vi "Register for Events (Cluster).vi"(8 "error in (no error)":errorcluster, 9 "Object":T1, 11 "JKI_Python_Server in":refnum<class "Server.lvclass">) -> (0 "error out":errorcluster, 1 "Python":T2, 3 "JKI_Python_Server out":refnum<class "Server.lvclass">)   [LabVIEW 2013, in "JKI_Python_Bridge_for_LV.lvlib" / "Server.lvclass"]
uses:
  Server.lvclass
  Type Definitions/Python Method Call - Event Registration.ctl
  Call/Call.lvclass
  Type Definitions/Public Events - Cluster.ctl
  CallHandler/PyObject.lvclass
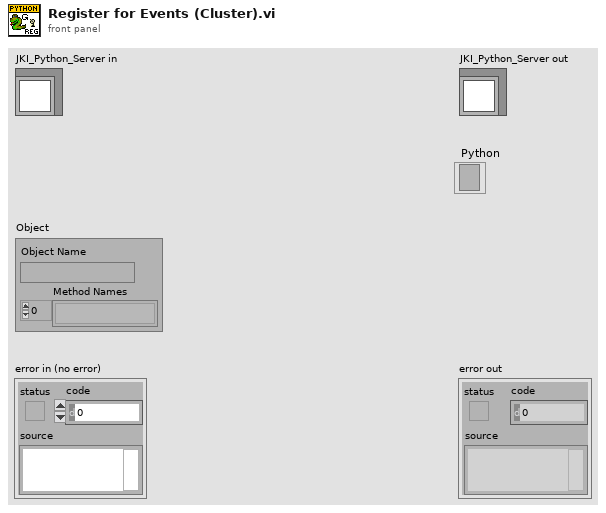
[diagram p1: front panel]
types:
  T1 = cluster{"Object Name":string, "Method Names":string[]}
  T2 = typedef "JKI_Python_Bridge_for_LV.lvlib/Server.lvclass/Python Method Call - Event Registration.ctl" = refnum<event-registration>
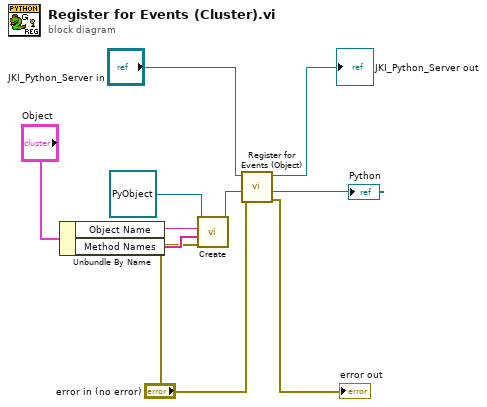
[diagram p0: block diagram]
diagram:
  n1 = Unbundle By Name("Object") -> ("Object Name"=w9:string, "Method Names"=w8:string[])
  n2 = call "Create.vi"("error in (no error)"="error in (no error)", "Method Names"=w8, "Object Name"=w9, "Node in"=refnum<class "PyObject.lvclass"> refnum) -> ("Node out"=w6:refnum<class "PyObject.lvclass">)  [unwired: 6 in, 1 out]
  n3 = call "Register for Events (Object).vi"("error in (no error)"="error in (no error)", "PyObject.lvclass"=w6, "JKI_Python_Server in"="JKI_Python_Server in") -> ("error out"=→"error out":errorcluster, "Python Event"=→"Python":T2, "JKI_Python_Server out"=→"JKI_Python_Server out":refnum<class "Server.lvclass">)  [unwired: 6 in]
